vi "X-Axis_Generator_morph.vi"   [LabVIEW 2019]
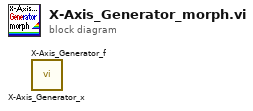
[diagram p0: block diagram]
diagram:
  n1 = call "X-Axis_Generator_x.vi"() -> ()  [unwired: 12 in, 8 out]
  n2 = call "X-Axis_Generator_f.vi"() -> ()  [unwired: 12 in, 8 out]
